vi "find_prime_number.vi"() -> ()   [LabVIEW 2021]
panel:
  out "is prime?":bool
  in  "Numeric":u64=1000000007
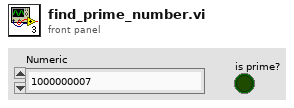
[diagram p1: front panel]
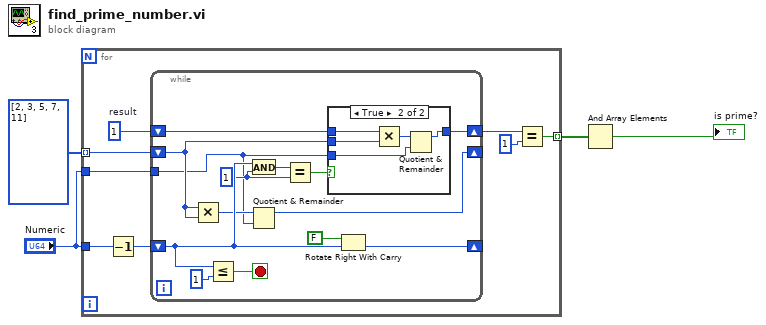
[diagram p0: block diagram]
diagram:
  n1 = for {
    tunnel: u64[] [2, 3, 5, 7, 11] -> [w6] mode=indexing
    tunnel: "Numeric" -> [w11]
    tunnel: "Numeric" -> [w9]
    tunnel: [w7] -> w2 mode=indexing
    w10 = 1  # result
    n2 = Decrement(x=w11) -> (x-1=w12:u64)
    n3 = while {
      shift-right: [w25] -> _
      shift-left: w12 -> [w22]
      shift-right: [w17] -> w5
      shift-left: w10 -> [w18]
      shift-right: [w13] -> _
      shift-left: w6 -> [w16]
      tunnel: w9 -> [w14]
      stop <- w23 stop-if-true
      w20 = u64 1 ("y")
      n4 = Multiply(x=w16, y=w16) -> (x*y=w15:u64)
      n5 = Less Or Equal?(x=w22, y=1) -> (x <= y?=w23:bool)
      n6 = And(x=w22, y=w20) -> (x .and. y?=w21:u64)
      n7 = Quotient & Remainder(x=w15, y=w14) -> (x-y*floor(x/y)=w13:u64)  [unwired: 1 out]
      n8 = Equal?(x=w21, y=w20) -> (x = y?=w19:bool)
      n9 = case shown="True" w19 {
        tunnel: w18 -> [w27 w32]
        tunnel: w16 -> [_ w31]
        tunnel: w14 -> [_ w29]
        tunnel: [w27 w28] -> w17
        frame False {
        }
        frame True {
          n10 = Multiply(x=w32, y=w31) -> (x*y=w30:u64)
          n11 = Quotient & Remainder(x=w30, y=w29) -> (x-y*floor(x/y)=w28:u64)  [unwired: 1 out]
        }
      }
      n12 = Rotate Right With Carry(2:w22, 3:FALSE ("carry")) -> (0:w25:u64)  [unwired: 1 out]
    }
    n13 = Equal?(x=w5, y=u64 1) -> (x = y?=w7:bool)
  }
  n14 = And Array Elements(Boolean array=w2) -> (logical AND=→"is prime?":bool)
